vi "子界面-查看某框和报告生成-第2版.vi"(0 "框号":dbl format="%#_13g", 1 "框组":T3(array[cluster]), 3 "反射图原始路径":path, 5 "预先配置的灰度阈值":dbl, 6 "穿透图原始路径":path, 7 "部位信息":string[](array[string])=["", "34.500000", "32.500000", "1121", "34", "54.955926", "分层类", "不合格", ""], 12 "产品规格":cluster{"产品长度（周长）（mm）":dbl, "产品宽度（母线长）（mm）":dbl}) -> (14 "弥散类检测结果":string[][](table), 19 "分层类检测结果":string[][](table))   [LabVIEW 2018]
uses:
  <vilib>/vision/NI_Vision_Development_Module.lvlib
panel:
  out "弥散缺陷个数":i32
  out "分层缺陷个数":i32
  out "合格？ 弥散类":string="fencengThreshold"
  out "合格？分层类":string="fencengThreshold"
  in  "stop":bool caption="停止"
  out "?":T1(plugin-control)
  out "Threshold Image":T1(plugin-control)
  out "Threshold Image":T1(plugin-control)
  out "Threshold Image":T1(plugin-control)
  out "反射图ROI的最大灰度值":sgl
  in  "灰度阈值设置":cluster{"下限":dbl, "下限":dbl}(slide)={"下限"=0.0, "下限"=65.10638427734375} scale=0.0..255.0
  in  "Tab Control":T2
  out "穿透ROI":T1(plugin-control)
  out "Threshold Image":T1(plugin-control)
  out "?":T1(plugin-control)
  out "?":T1(plugin-control)
  out "Threshold Image":T1(plugin-control)
  out "Threshold Image":T1(plugin-control)
  out "弥散测量结果":dbl[][](array[numeric]) format="%.2f"
  in  "分隔符（'\\'代码显示）":string="\t"
  in  "格式字符串":string="%f"
  out "?":string
  out "面积 (pixels)":i32
  in  "格式字符串 2":string="%f"
  in  "分隔符（'\\'代码显示）":string="\t"
  out "分层测量结果":dbl[][](array[numeric]) format="%.2f"
  out "缺陷分类的临界值":sgl format="%#.3f"
  # "所选区域信息"
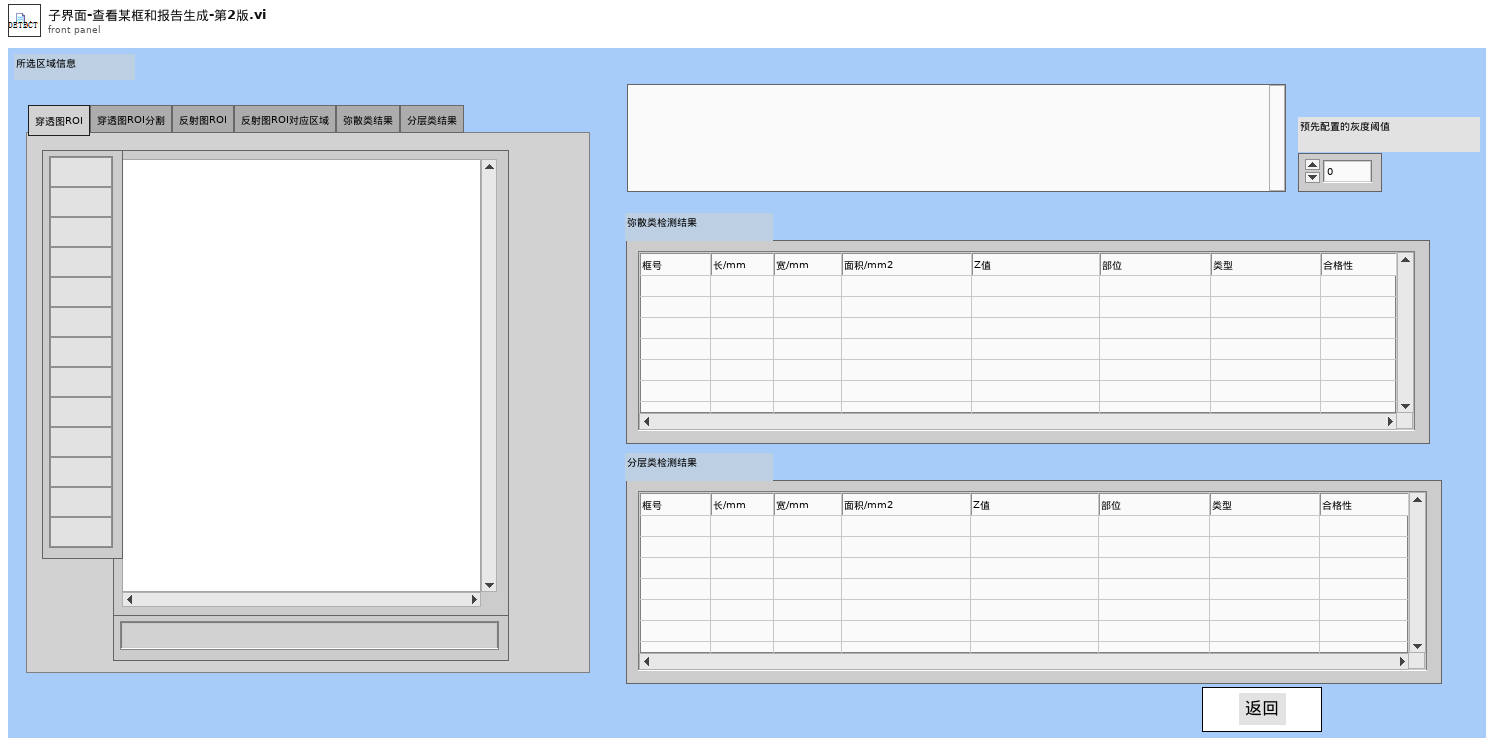
[diagram p1: front panel]
types:
  T1 = typedef "IMAQ Image.ctl" = refnum<image>
  T2 = typedef "控件 1.ctl" = enum32{"穿透图ROI", "穿透图ROI分割", "反射图ROI", "反射图ROI对应区域", "弥散类结果", "分层类结果"}
  T3 = cluster{"Global Rectangle":i32[], "Contours":cluster{"Contour Type":u32, "ROI Type":u32, "Points":i32[]}[]}[]
  T4 = typedef "Image Type" = u32
  T5 = typedef "Particle Parameters" = i32
  T6 = cluster{"Measurement Parameter":T5, "Range Lower Value":dbl, "Range Upper Value":dbl, "Range":bool, "Measurement Type":bool}[]
  T7 = cluster{"Global Rectangle":i32[], "Contours":cluster{"Contour Type":u32, "ROI Type":u32, "Points":i32[]}[]}
  T8 = cluster{"histogram":u32[], "Minimal Value":sgl, "Maximal Value":sgl, "Starting Value":sgl, "Interval Width":sgl, "Mean Value":sgl, "Standard  Variation":sgl, "Area (pixels)":i32}
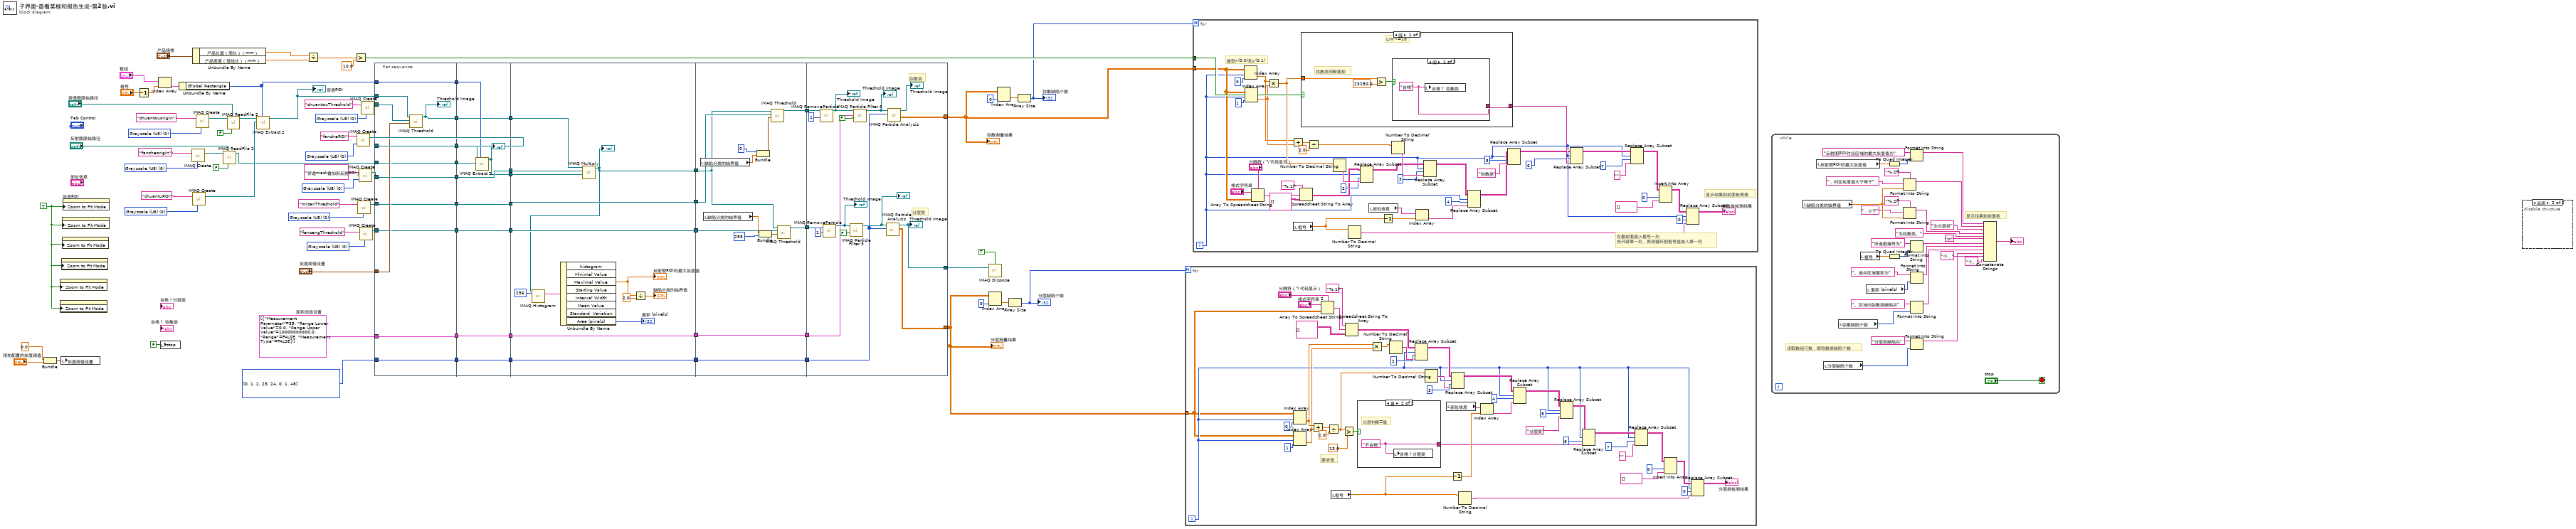
[diagram p0: block diagram]
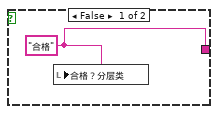
[diagram p2: hidden frame]
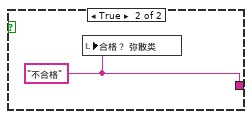
[diagram p3: hidden frame]
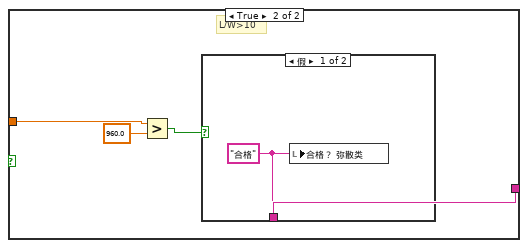
[diagram p4: hidden frame]
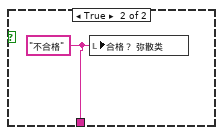
[diagram p5: hidden frame]
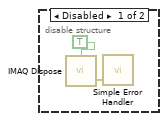
[diagram p6: hidden frame]
diagram:
  w48 = T4 0 items=["Grayscale (U8)", "Grayscale (I16)", "Grayscale (SGL)", "Complex (CSG)", "RGB (U32)", "HSL (U32)", "RGB (U64)", "Grayscale (U16)"] ("Image Type")
  w49 = T4 0 items=["Grayscale (U8)", "Grayscale (I16)", "Grayscale (SGL)", "Complex (CSG)", "RGB (U32)", "HSL (U32)", "RGB (U64)", "Grayscale (U16)"] ("Image Type")
  w50 = T4 0 items=["Grayscale (U8)", "Grayscale (I16)", "Grayscale (SGL)", "Complex (CSG)", "RGB (U32)", "HSL (U32)", "RGB (U64)", "Grayscale (U16)"] ("Image Type")
  w54 = T4 0 items=["Grayscale (U8)", "Grayscale (I16)", "Grayscale (SGL)", "Complex (CSG)", "RGB (U32)", "HSL (U32)", "RGB (U64)", "Grayscale (U16)"] ("Image Type")
  w58 = T4 0 items=["Grayscale (U8)", "Grayscale (I16)", "Grayscale (SGL)", "Complex (CSG)", "RGB (U32)", "HSL (U32)", "RGB (U64)", "Grayscale (U16)"] ("Image Type")
  w6 = i32[] [0, 1, 2, 23, 24, 0, 1, 48] items=["Bounding Rect Width", "Bounding Rect Height", "Area"] ("Pixel Measurements")
  w11 = T6 [{"Measurement Parameter"=35, "Range Lower Value"=0.0, "Range Upper Value"=10000000000.0, "Range"=FALSE, "Measurement Type"=FALSE}]  # 面积阈值设置
  w72 = T4 0 items=["Grayscale (U8)", "Grayscale (I16)", "Grayscale (SGL)", "Complex (CSG)", "RGB (U32)", "HSL (U32)", "RGB (U64)", "Grayscale (U16)"] ("Image Type")
  w41 = T4 0 items=["Grayscale (U8)", "Grayscale (I16)", "Grayscale (SGL)", "Complex (CSG)", "RGB (U32)", "HSL (U32)", "RGB (U64)", "Grayscale (U16)"] ("Image Type")
  w76 = T4 0 items=["Grayscale (U8)", "Grayscale (I16)", "Grayscale (SGL)", "Complex (CSG)", "RGB (U32)", "HSL (U32)", "RGB (U64)", "Grayscale (U16)"] ("Image Type")
  w85 = TRUE ("Zoom to Fit Mode")
  n1 = Bundle(0.0, "预先配置的灰度阈值"="预先配置的灰度阈值") -> (w83:cluster{dbl, "预先配置的灰度阈值":dbl})  [unwired: 1 in]
  n2 = property class="ImageControl"("Zoom to Fit Mode"=w85) -> ()  [unwired: 2 in, 2 out]
  n3 = property class="ImageControl"("Zoom to Fit Mode"=w85) -> ()  [unwired: 2 in, 2 out]
  n4 = local write "灰度阈值设置"(w83) -> ()
  n5 = property class="ImageControl"("Zoom to Fit Mode"=w85) -> ()  [unwired: 2 in, 2 out]
  n6 = property class="ImageControl"("Zoom to Fit Mode"=w85) -> ()  [unwired: 2 in, 2 out]
  n7 = property class="ImageControl"("Zoom to Fit Mode"=w85) -> ()  [unwired: 2 in, 2 out]
  n8 = property on="穿透ROI" class="ImageControl"("Zoom to Fit Mode"=w85) -> ()  [unwired: 2 in, 2 out]
  n9 = Decrement(x="框号") -> (x-1=w78:dbl)
  n10 = Index Array(array="框组", index=w78) -> (element=w79:T7)
  n11 = local write "stop"(FALSE ("stop")) -> ()
  n12 = Unbundle By Name(w79) -> ("Global Rectangle"=w40:i32[])
  n13 = call "IMAQ Create"("Image Name"="fansheorigin", "Image Type"=w54) -> ("New Image"=w53:T1)  [unwired: 3 in, 1 out]
  n14 = call "IMAQ Create"("Image Name"="chuantuROI", "Image Type"=w58) -> ("New Image"=w57:T1)  [unwired: 3 in, 1 out]
  n15 = Unbundle By Name("产品规格") -> ("产品长度（周长）（mm）"=w66:dbl, "产品宽度（母线长）（mm）"=w65:dbl)
  n16 = call "IMAQ Create"("Image Name"="chuantouorigin", "Image Type"=w76) -> ("New Image"=w60:T1)  [unwired: 3 in, 1 out]
  n17 = call "IMAQ ReadFile 2"("Use File Path Image Type"=FALSE, "File Path"="反射图原始路径", "Image"=w53) -> ("Image Out"=w35:T1)  [unwired: 4 in, 4 out]
  n18 = call "IMAQ ReadFile 2"("Use File Path Image Type"=FALSE, "File Path"="穿透图原始路径", "Image"=w60) -> ("Image Out"=w61:T1)  [unwired: 4 in, 4 out]
  n19 = call "IMAQ Extract 2"("Optional Rectangle"=w40, "Image Dst"=w57, "Image Src"=w61) -> ("Image Dst Out"=w38:T1)  [unwired: 7 in, 1 out]
  "穿透ROI" <- w38
  n20 = Divide(x=w66, y=w65) -> (x/y=w69:dbl)
  n21 = Greater?(x=w69, y=10.0) -> (0:w64:bool)
  n22 = call "IMAQ Create"("Image Name"="fansheROI", "Image Type"=w41) -> ("New Image"=w36:T1)  [unwired: 3 in, 1 out]
  n23 = call "IMAQ Create"("Image Name"="misanThreshold", "Image Type"=w48) -> ("New Image"=w22:T1)  [unwired: 3 in, 1 out]
  n24 = call "IMAQ Create"("Image Name"="穿透mask叠加到反射ROI上", "Image Type"=w72) -> ("New Image"=w30:T1)  [unwired: 3 in, 1 out]
  n25 = call "IMAQ Create"("Image Name"="fencengThreshold", "Image Type"=w49) -> ("New Image"=w20:T1)  [unwired: 3 in, 1 out]
  n26 = call "IMAQ Create"("Image Name"="chuantouThreshold", "Image Type"=w50) -> ("New Image"=w39:T1)  [unwired: 3 in, 1 out]
  n27 = flat-sequence {
    tunnel: w40 -> [w97]
    tunnel: w39 -> [w96]
    tunnel: w38 -> [w95]
    tunnel: "灰度阈值设置" -> [w94]
    tunnel: w36 -> [w93]
    tunnel: w35 -> [w92]
    tunnel: [w97] -> w34
    tunnel: [w93] -> w33
    tunnel: [w92] -> w32
    tunnel: [w91] -> w31
    tunnel: w30 -> [w91]
    tunnel: [w90] -> w27
    tunnel: w22 -> [w89]
    tunnel: [w89] -> w24
    tunnel: [w88] -> w21
    tunnel: w20 -> [w88]
    tunnel: [w87] -> w12
    tunnel: w11 -> [w87]
    tunnel: [w86] -> w7
    tunnel: w6 -> [w86]
    tunnel: w34 -> [w107]
    tunnel: w33 -> [w105]
    tunnel: w32 -> [w106]
    tunnel: w31 -> [w104]
    tunnel: [w104] -> w29
    tunnel: [w103] -> w28
    tunnel: w27 -> [w103]
    tunnel: [w102] -> w26
    tunnel: w24 -> [w101]
    tunnel: [w101] -> w23
    tunnel: w21 -> [w100]
    tunnel: [w100] -> w19
    tunnel: w12 -> [w99]
    tunnel: [w99] -> w10
    tunnel: w7 -> [w98]
    tunnel: [w98] -> w5
    tunnel: w29 -> [w121]
    tunnel: w28 -> [w120]
    tunnel: w26 -> [w119]
    tunnel: [w118] -> w25
    tunnel: w23 -> [w118]
    tunnel: w19 -> [w117]
    tunnel: [w117] -> w18
    tunnel: [w110] -> w17
    tunnel: w10 -> [w109]
    tunnel: [w109] -> w9
    tunnel: w5 -> [w108]
    tunnel: [w108] -> w4
    tunnel: w25 -> [w129]
    tunnel: w18 -> [w128]
    tunnel: w17 -> [w127]
    tunnel: [w126] -> w14
    tunnel: [w125] -> w13
    tunnel: w9 -> [w124]
    tunnel: [w124] -> w8
    tunnel: w4 -> [w123]
    tunnel: [w123] -> w3
    tunnel: [w145] -> w16
    tunnel: [w140] -> w1
    tunnel: [w139] -> w15
    tunnel: w14 -> [w138]
    tunnel: w13 -> [w137]
    tunnel: w8 -> [w136]
    tunnel: w3 -> [w135]
    frame #0 {
      n28 = call "IMAQ Threshold"("Range"=w94, "Image Dst"=w96, "Image Src"=w95) -> ("Image Dst Out"=w90:T1)  [unwired: 3 in, 5 out]
      "Threshold Image" <- w90
    }
    frame #1 {
      n29 = call "IMAQ Extract 2"("Optional Rectangle"=w107, "Image Dst"=w106, "Image Src"=w105) -> ("Image Dst Out"=w102:T1)  [unwired: 7 in, 1 out]
      "?" <- w102
    }
    frame #2 {
      n30 = call "IMAQ Multiply"("Image Src A"=w120, "Image Dst"=w121, "Image Src B"=w119) -> ("Image Dst Out"=w110:T1)  [unwired: 4 in, 1 out]
      "?" <- w110
      n31 = call "IMAQ Histogram"("Number of Classes"=256, "Image"=w110) -> ("Histogram Report"=w113:T8)  [unwired: 8 in, 1 out]
      n32 = Unbundle By Name(w113) -> ("Maximal Value"=w115:sgl, "Area (pixels)"=→"面积 (pixels)":i32)  [unwired: 6 out]
      "反射图ROI的最大灰度值" <- w115
      n33 = Divide(x=w115, y=sgl 2.0) -> (x/y=→"缺陷分类的临界值":sgl)
    }
    frame #3 {
      n34 = local read "缺陷分类的临界值"() -> (w134:sgl)
      n35 = local read "缺陷分类的临界值"() -> (w132:sgl)
      n36 = Bundle(0, "缺陷分类的临界值"=w134) -> (w122:cluster{i32, "缺陷分类的临界值":sgl})  [unwired: 1 in]
      n37 = Bundle("缺陷分类的临界值"=w132, 255) -> (w131:cluster{"缺陷分类的临界值":sgl, i32})  [unwired: 1 in]
      n38 = call "IMAQ Threshold"("Range"=w122, "Image Dst"=w129, "Image Src"=w127) -> ("Image Dst Out"=w125:T1)  [unwired: 3 in, 5 out]
      n39 = call "IMAQ Threshold"("Range"=w131, "Image Dst"=w128, "Image Src"=w127) -> ("Image Dst Out"=w126:T1)  [unwired: 3 in, 5 out]
    }
    frame #4 {
      # "分层类"
      # "弥散类"
      n40 = call "IMAQ RemoveParticle"("Number of Erosion"=1, "Image Src"=w137) -> ("Image Dst Out"=w148:T1)  [unwired: 8 in, 1 out]
      "Threshold Image" <- w148
      n41 = call "IMAQ RemoveParticle"("Number of Erosion"=1, "Image Src"=w138) -> ("Image Dst Out"=w143:T1)  [unwired: 8 in, 1 out]
      "Threshold Image" <- w143
      n42 = call "IMAQ Particle Filter 3"("Image Src"=w143, "Keep/Remove Particles (F)"=FALSE) -> ("Image Dst Out"=w144:T1)  [unwired: 11 in, 2 out]
      "?" <- w144
      n43 = call "IMAQ Particle Filter 3"("Image Src"=w148, "Selection Values"=w136, "Keep/Remove Particles (F)"=FALSE) -> ("Image Dst Out"=w149:T1)  [unwired: 10 in, 2 out]
      "Threshold Image" <- w149
      n44 = call "IMAQ Particle Analysis"("Pixel Measurements"=w135, "Image"=w144) -> ("Particle Measurements (Pixels)"=w140:dbl[][], "Image Out (duplicate)"=w139:T1)  [unwired: 4 in, 4 out]
      "Threshold Image" <- w139
      n45 = call "IMAQ Particle Analysis"("Pixel Measurements"=w135, "Image"=w149) -> ("Particle Measurements (Real-World)"=w145:dbl[][], "Image Out (duplicate)"=→"Threshold Image":T1)  [unwired: 4 in, 4 out]
    }
  }
  n46 = call "IMAQ Dispose"("All Images? (No)"=TRUE, "Image"=w15) -> ()  [unwired: 4 in, 1 out]
  n47 = Index Array(array=w1, index (col)=0 ("禁用的索引 (列)")) -> (element=w46:dbl[])  [unwired: 1 in]
  n48 = Index Array(array=w16, index (col)=0 ("禁用的索引 (列)")) -> (element=w44:dbl[])  [unwired: 1 in]
  n49 = Array Size(array=w46) -> (size(s)=w2:i32)
  "分层缺陷个数" <- w2
  n50 = Array Size(array=w44) -> (size(s)=w63:i32)
  "弥散缺陷个数" <- w63
  n51 = for {
    N: w2 -> [_]
    tunnel: w1 -> [w151]
    i -> [w154]
    # "要求值"
    n52 = Index Array(array=w151, index (row)=w154, index (col)=0 ("禁用的索引 (列)")) -> (element=w168:dbl)
    n53 = Index Array(array=w151, index (row)=w154, index (col)=1 ("禁用的索引 (列)")) -> (element=w167:dbl)
    n54 = Add(x=w168, y=w167) -> (x+y=w194:dbl)
    n55 = Array To Spreadsheet String(delimiter (Tab)="分隔符（'\\'代码显示）", array=w151, 3:"格式字符串 2") -> (spreadsheet string=w193:string)
    n56 = Divide(x=w194, y=2.0) -> (x/y=w182:dbl)
    n57 = local read "框号"() -> (w152:dbl)
    n58 = Greater?(x=w182, y=13.0) -> (0:w195:bool)
    n59 = Spreadsheet String To Array(format string="%.1f", spreadsheet string=w193, array type (2D Dbl)=string[][] [] ("Array")) -> (array=w179:string[][])  [unwired: 1 in]
    n60 = case shown="真" w195 {
      tunnel: [w196 w197] -> w161
      frame False {
        w196 = "合格" ("合格？")
        n61 = local write "合格？分层类"(w196) -> ()
      }
      frame True {
        w197 = "不合格" ("合格？")
        # "分层判断Z值"
        n62 = local write "合格？分层类"(w197) -> ()
      }
    }
    n63 = Multiply(x=w168, y=w167) -> (x*y=w180:dbl)
    n64 = Number To Decimal String(number=w180) -> (decimal integer string=w166:string)  [unwired: 1 in]
    n65 = Replace Array Subset(array=w179, new element=w166, index (row)=w154, index (col)=2 ("禁用的索引 (列)")) -> (w175:string[][])
    n66 = Number To Decimal String(number=w182) -> (decimal integer string=w165:string)  [unwired: 1 in]
    n67 = local read "部位信息"() -> (w172:string[])
    n68 = Decrement(x=w152) -> (x-1=w171:dbl)
    n69 = Replace Array Subset(array=w175, new element=w165, index (row)=w154, index (col)=3 ("禁用的索引 (列)")) -> (w170:string[][])
    n70 = Number To Decimal String(number=w152) -> (decimal integer string=w153:string)  [unwired: 1 in]
    n71 = Index Array(array=w172, index=w171) -> (element=w164:string)
    n72 = Replace Array Subset(array=w170, new element=w164, index (row)=w154, index (col)=4 ("禁用的索引 (列)")) -> (w169:string[][])
    n73 = Replace Array Subset(array=w169, new element="分层类" ("新元素/子数组"), index (row)=w154, index (col)=5 ("禁用的索引 (列)")) -> (w174:string[][])
    n74 = Replace Array Subset(array=w174, new element=w161, index (row)=w154, index (col)=6 ("禁用的索引 (列)")) -> (w177:string[][])
    n75 = Replace Array Subset(array=w177, new element="" ("新元素/子数组"), index (row)=w154, index (col)=7 ("禁用的索引 (列)")) -> (w156:string[][])
    n76 = Insert Into Array(array=w156, index (col)=0 ("禁用的索引 (列)"), new element=string[] [] ("新元素/子数组")) -> (w158:string[][])  [unwired: 1 in]
    n77 = Replace Array Subset(array=w158, new element=w153, index (row)=w154, index (col)=0 ("禁用的索引 (列)")) -> (→"分层类检测结果":string[][])
  }
  n78 = for {
    N: w63 -> [_]
    tunnel: w64 -> [w241]
    tunnel: w16 -> [w240]
    i -> [w201]
    # "在最前面插入框号一列\n先开辟第一列，再用循环把框号值放入第一列"
    # "提取x(0,0)和y(0,1)"
    # "显示结果到前面板表格"
    n79 = Index Array(array=w240, index (row)=w201, index (col)=0 ("禁用的索引 (列)")) -> (element=w224:dbl)
    n80 = Index Array(array=w240, index (row)=w201, index (col)=1 ("禁用的索引 (列)")) -> (element=w223:dbl)
    n81 = Array To Spreadsheet String(delimiter (Tab)="分隔符（'\\'代码显示）", array=w240, 3:"格式字符串") -> (spreadsheet string=w238:string)
    n82 = Multiply(x=w224, y=w223) -> (x*y=w227:dbl)
    n83 = Add(x=w224, y=w223) -> (x+y=w226:dbl)
    n84 = local read "框号"() -> (w205:dbl)
    n85 = Spreadsheet String To Array(format string="%.1f", spreadsheet string=w238, array type (2D Dbl)=string[][] [] ("Array")) -> (array=w215:string[][])  [unwired: 1 in]
    n86 = case shown="假" w241 {
      tunnel: w227 -> [w244 w251]
      tunnel: [w242 w248] -> w239
      frame False {
        # "弥散类判断面积"
        # "L/W<=10"
        n87 = Greater?(x=w244, y=23250.0) -> (0:w243:bool)
        n88 = case shown="假" w243 {
          tunnel: [w246 w247] -> w242
          frame False {
            w246 = "合格" ("合格？")
            n89 = local write "合格？ 弥散类"(w246) -> ()
          }
          frame True {
            w247 = "不合格" ("合格？")
            n90 = local write "合格？ 弥散类"(w247) -> ()
          }
        }
      }
      frame True {
        # "L/W>10"
        n91 = Greater?(x=w251, y=960.0) -> (0:w249:bool)
        n92 = case shown="假" w249 {
          tunnel: [w252 w253] -> w248
          frame False {
            w252 = "合格" ("合格？")
            n93 = local write "合格？ 弥散类"(w252) -> ()
          }
          frame True {
            w253 = "不合格" ("合格？")
            n94 = local write "合格？ 弥散类"(w253) -> ()
          }
        }
      }
    }
    n95 = Divide(x=w226, y=2.0) -> (x/y=w220:dbl)
    n96 = Number To Decimal String(number=w227) -> (decimal integer string=w229:string)  [unwired: 1 in]
    n97 = Number To Decimal String(number=w205) -> (decimal integer string=w199:string)  [unwired: 1 in]
    n98 = Replace Array Subset(array=w215, new element=w229, index (row)=w201, index (col)=2 ("禁用的索引 (列)")) -> (w214:string[][])
    n99 = local read "部位信息"() -> (w210:string[])
    n100 = Decrement(x=w205) -> (x-1=w209:dbl)
    n101 = Number To Decimal String(number=w220) -> (decimal integer string=w222:string)  [unwired: 1 in]
    n102 = Index Array(array=w210, index=w209) -> (element=w208:string)
    n103 = Replace Array Subset(array=w214, new element=w222, index (row)=w201, index (col)=3 ("禁用的索引 (列)")) -> (w207:string[][])
    n104 = Replace Array Subset(array=w207, new element=w208, index (row)=w201, index (col)=4 ("禁用的索引 (列)")) -> (w206:string[][])
    n105 = Replace Array Subset(array=w206, new element="弥散类" ("新元素/子数组"), index (row)=w201, index (col)=5 ("禁用的索引 (列)")) -> (w213:string[][])
    n106 = Replace Array Subset(array=w213, new element=w239, index (row)=w201, index (col)=6 ("禁用的索引 (列)")) -> (w212:string[][])
    n107 = Replace Array Subset(array=w212, new element="" ("新元素/子数组"), index (row)=w201, index (col)=7 ("禁用的索引 (列)")) -> (w204:string[][])
    n108 = Insert Into Array(array=w204, index (col)=0 ("禁用的索引 (列)"), new element=string[] [] ("新元素/子数组")) -> (w202:string[][])  [unwired: 1 in]
    n109 = Replace Array Subset(array=w202, new element=w199, index (row)=w201, index (col)=0 ("禁用的索引 (列)")) -> (→"弥散类检测结果":string[][])
  }
  n110 = while {
    stop <- "stop" stop-if-true
    # "显示结果到前面板"
    # "读取数组行数，即弥散类缺陷个数"
    n111 = local read "缺陷分类的临界值"() -> (w284:sgl)
    n112 = local read "反射图ROI的最大灰度值"() -> (w276:sgl)
    n113 = local read "分层缺陷个数"() -> (w255:i32)
    n114 = local read "弥散缺陷个数"() -> (w254:i32)
    n115 = local read "框号"() -> (w272:dbl)
    n116 = local read "面积 (pixels)"() -> (w275:i32)
    n117 = To Quad Integer(1:w276) -> (0:w277:i64)
    n118 = To Quad Integer(1:w272) -> (0:w273:i64)
    n119 = Format Into String(format string="%.2f" ("格式字符串"), initial string="，判定灰度值大于等于" ("初始字符串"), w284) -> (resulting string=w279:string)  [unwired: 1 in, 1 out]
    n120 = Format Into String(format string="%.2f" ("格式字符串"), initial string="，小于" ("初始字符串"), w284) -> (resulting string=w278:string)  [unwired: 1 in, 1 out]
    n121 = Format Into String(initial string="反射图ROI对应区域的最大灰度值为" ("初始字符串"), w277) -> (resulting string=w280:string)  [unwired: 2 in, 1 out]
    n122 = Format Into String(initial string="所选框编号为" ("初始字符串"), w273) -> (resulting string=w271:string)  [unwired: 2 in, 1 out]
    n123 = Format Into String(initial string="。选中区域面积为" ("字符串"), w275) -> (resulting string=w281:string)  [unwired: 2 in, 1 out]
    n124 = Format Into String(initial string="。区域内弥散类缺陷共" ("初始字符串"), w254) -> (resulting string=w282:string)  [unwired: 2 in, 1 out]
    n125 = Format Into String(initial string="分层类缺陷共" ("初始字符串"), w255) -> (resulting string=w283:string)  [unwired: 2 in, 1 out]
    n126 = Concatenate Strings(w280, w279, "为分层类" ("初始字符串"), w278, "为弥散类。" ("初始字符串"), "\n", w271, w281, w282, "个，" ("字符串"), w283, "个。" ("字符串")) -> (→"?":string)
  }
  n127 = disable-structure shown="启用" {
    frame Disabled {
      n128 = call "IMAQ Dispose"("All Images? (No)"=TRUE) -> ("error out"=w286:errorcluster)  [unwired: 5 in]
      n129 = call <vilib>:"Simple Error Handler.vi"("error in (no error)"=w286) -> ()  [unwired: 4 in, 5 out]
    }
    frame Enabled {
    }
  }
  "分层测量结果" <- w1
  "弥散测量结果" <- w16
